vi "Dan-ReadLidar.vi"(10 "Raphael_Offsets":T1={"x_offset"=2000, "y_offset"=-420, "z_offset"=1000, "Theta_z"=0.0, "Theta_y"=22.0} {"Theta_y" format="%.10g"; "Theta_z" format="%.10g"}, 11 "Leonardo_Offsets":T1={"x_offset"=2000, "y_offset"=420, "z_offset"=1000, "Theta_z"=0.0, "Theta_y"=12.0} {"Theta_y" format="%.10g"; "Theta_z" format="%.10g"}) -> ()   [LabVIEW 2010]
doc: "ReadLidars.vi: sets the LIDARS to stream continously, then reads them and sends a stream of (x,y,z) local coordinates of the last read LIDAR points to the PC."
uses:
  Type Defs/LidarOffsets.ctl
  <vilib>/eio/EIOMethodNode/EIOMethodNode.xnode
  <vilib>/rvi/eio/nirviEIOMethodImplementation/nirviEIOMethodImplementation.xnode
  <vilib>/rvi/eio/common/nirviEmuClasses.ctl
  <vilib>/rvi/eio/common/nirviEmuTemplateMethod_noerrors.vi
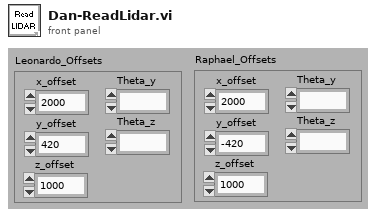
[diagram p1: front panel]
types:
  T1 = typedef "LidarOffsets.ctl" = cluster{"x_offset":i16, "y_offset":i16, "z_offset":i16, "Theta_z":fxp<+/-,16,9>, "Theta_y":fxp<+/-,16,9>}
  T2 = typedef "nirviEmuClasses.ctl" = enum16{"IO Read", "IO Write", "Method", "Property Read", "Property Write"}
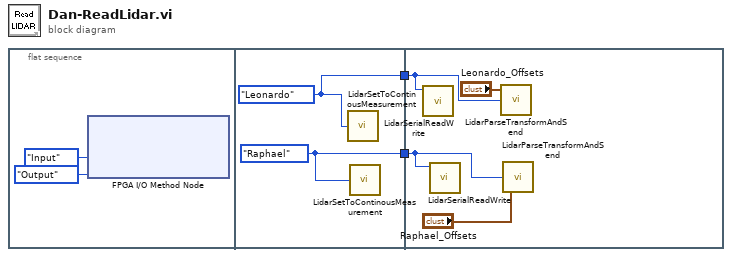
[diagram p0: block diagram]
diagram:
  n1 = flat-sequence {
    tunnel: [w19] -> w2
    tunnel: [w18] -> w1
    tunnel: w2 -> [w23]
    tunnel: w1 -> [w22]
    frame #0 {
      n2 = xnode "FPGA I/O Method Node"("DIO 7:4"=enum8{"No Change", "Input", "Output"}."Input", "DIO 3:0"=enum8{"No Change", "Input", "Output"}."Output") -> ()  [unwired: 1 in, 1 out]
    }
    frame #1 {
      w18 = enum16{"Raphael", "Leonardo"}."Leonardo" ("SelectLIDAR 2")
      w19 = enum16{"Raphael", "Leonardo"}."Raphael" ("SelectLIDAR")
      n3 = call "LidarSetToContinousMeasurement.vi"("SelectLIDAR"=w18) -> ()  [unwired: 1 in]
      n4 = call "LidarSetToContinousMeasurement.vi"("SelectLIDAR"=w19) -> ()  [unwired: 1 in]
    }
    frame #2 {
      n5 = call "LidarSerialReadWrite.vi"("SelectLIDAR"=w22) -> ()  [unwired: 11 in]
      n6 = call "LidarSerialReadWrite.vi"("SelectLIDAR"=w23) -> ()  [unwired: 11 in]
      n7 = call "LidarParseTransformAndSend.vi"("SelectLIDAR"=w22, "Leonardo_Offsets"="Leonardo_Offsets") -> ()  [unwired: 1 in, 1 out]
      n8 = call "LidarParseTransformAndSend.vi"("Raphael_Offsets"="Raphael_Offsets", "SelectLIDAR"=w23) -> ()  [unwired: 1 in, 1 out]
    }
  }
